vi "Mixed Signal Graph.vi"() -> ()   [LabVIEW 2023]
doc: "This example shows how to use the Mixed Signal Graph to display various types of signals in a single graph indicator on the front panel."
uses:
  <vilib>/Waveform/DWDTOps.llb/Digital Pattern Generator (Random).vi
panel:
  out "Mixed Signal Graph":T1(graph)
  # "Overview: Demonstrates the use of the Mixed Signal Graph to display different types of signals in a single graph.\nInstructions:\n1. Run the VI. Notice that various types of signals are displayed within different plot areas, or Groups.\n2. Right-click the plot area and select Add Plot Area.\n3. Drag any existing plot in the tree to the new group. Note that analog and digital signals cannot be displayed within the same plot area."
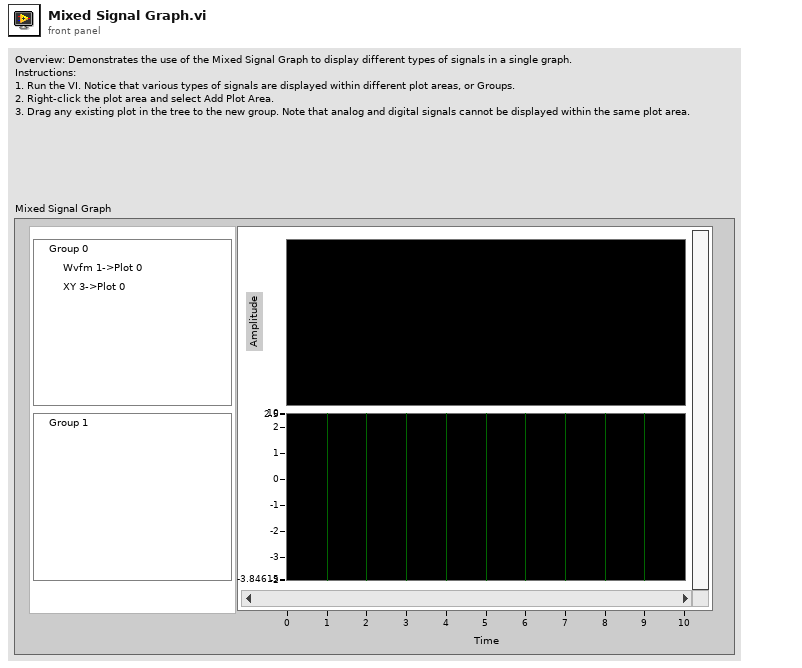
[diagram p1: front panel]
types:
  T1 = cluster{"Sine":dynamicdata, dbl[], "digital waveform":digitalwaveform, cluster{dbl[], dbl[]}}
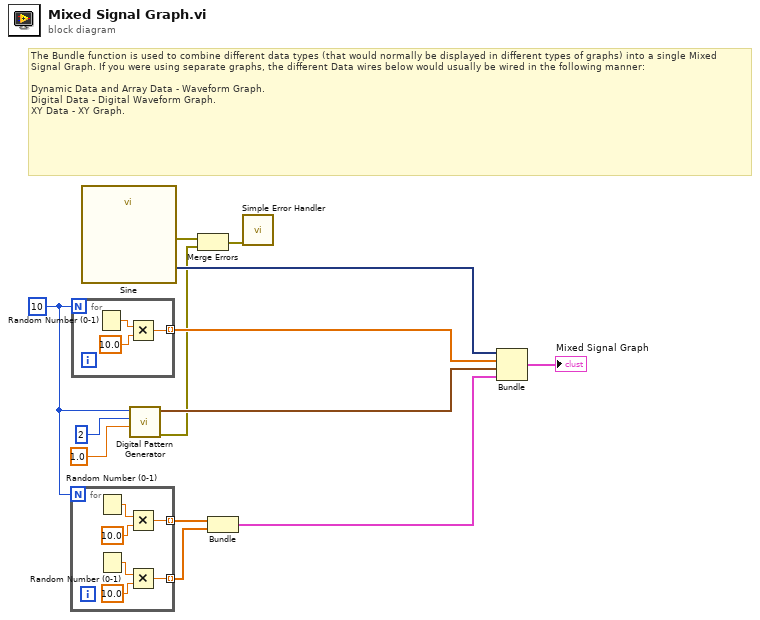
[diagram p0: block diagram]
diagram:
  w4 = 10
  # "The Bundle function is used to combine different data types (that would normally be displayed in different types of graphs) into a single Mixed Signal Graph. If you were using separate graphs, the different Data wires below would usually be wired in the following manner:\n\nDynamic Data and Array Data - Waveform Graph.\nDigital Data - Digital Waveform Graph.\nXY Data - XY Graph."
  n1 = for {
    N: w4 -> [_]
    tunnel: [w18] -> w8 mode=indexing
    tunnel: [w14] -> w7 mode=indexing
    n2 = Random Number (0-1)() -> (number: 0 to 1=w19:dbl)
    n3 = Random Number (0-1)() -> (number: 0 to 1=w15:dbl)
    n4 = Multiply(x=w19, y=10.0) -> (x*y=w18:dbl)
    n5 = Multiply(x=w15, y=10.0) -> (x*y=w14:dbl)
  }
  n6 = for {
    N: w4 -> [_]
    tunnel: [w21] -> w10 mode=indexing
    n7 = Random Number (0-1)() -> (number: 0 to 1=w22:dbl)
    n8 = Multiply(x=w22, y=10.0) -> (x*y=w21:dbl)
  }
  n9 = call "Sine"() -> ("Sine"=w11:dynamicdata, "error out"=w3:errorcluster)  [unwired: 14 in]
  n10 = call-poly <vilib>:"Digital Pattern Generator.vi"("sample rate"=1.0, "number of signals"=u32 2, "number of samples"=w4) -> ("error out"=w2:errorcluster, "digital waveform"=w9:digitalwaveform)  [unwired: 7 in]
  n11 = Merge Errors(w3, w2) -> (w1:errorcluster)
  n12 = Bundle(w8, w7) -> (w6:cluster{dbl[], dbl[]})  [unwired: 1 in]
  n13 = call <vilib>:"Simple Error Handler.vi"("error in (no error)"=w1) -> ()  [unwired: 4 in, 5 out]
  n14 = Bundle "Bundle"("Sine"=w11, w10, "digital waveform"=w9, w6) -> (→"Mixed Signal Graph":T1)  [unwired: 1 in]
